vi "FindInstruments.vi"(8 "error in (no error)":errorcluster, 10 "InstrumentData":T2, 11 "Jiaxin_Stepper_Controller in":refnum<class "Jiaxin_Stepper_Controller.lvclass">) -> (0 "error out":errorcluster, 3 "Jiaxin_Stepper_Controller out":refnum<class "Jiaxin_Stepper_Controller.lvclass">)   [LabVIEW 2023, in "Jiaxin_Stepper_Controller.lvlib" / "Jiaxin_Stepper_Controller.lvclass"]
uses:
  Jiaxin_Stepper_Controller.lvclass
  typedefs/instrumentType.ctl
  typedefs/typedefs.lvlib
  <vilib>/ActorFramework/Message Enqueuer/Message Enqueuer.lvclass
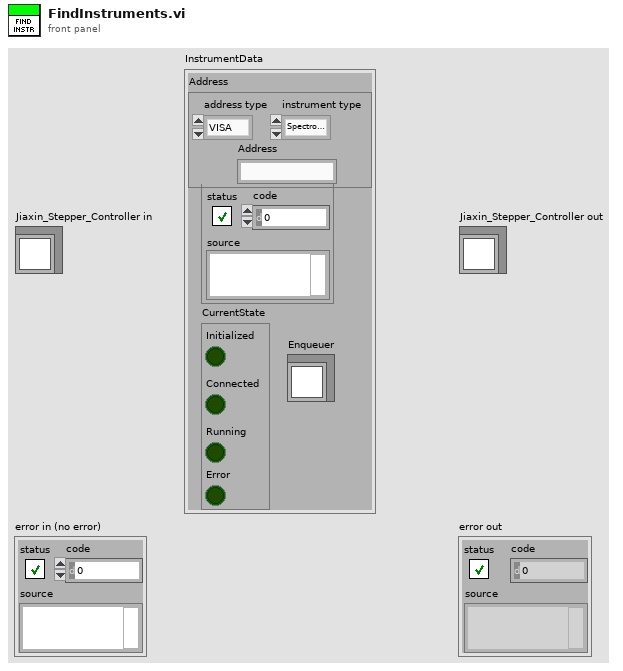
[diagram p1: front panel]
types:
  T1 = typedef "typedefs.lvlib/instrumentType.ctl" = enum16{"Spectrometer", "Camera", "Stepper", "Piezo"}
  T2 = cluster{"Instr Error":errorcluster, "Address":cluster{"address type":enum16{"VISA", "Index"}, "Address":string, "instrument type":T1}, "CurrentState":cluster{"Initialized":bool, "Connected":bool, "Running":bool, "Error":bool}, "Enqueuer":refnum<class "Message Enqueuer.lvclass">}
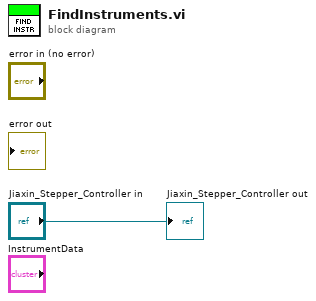
[diagram p0: block diagram]
diagram:
  "Jiaxin_Stepper_Controller out" <- "Jiaxin_Stepper_Controller in"
